vi "Read PID Kp.vi"(8 "error in (no error)":errorcluster, 10 "node":u8, 11 "ProPar in":refnum<class "PL Bronkhorst ProPar.lvclass">) -> (0 "error out":errorcluster, 2 "PID Kp":sgl, 3 "ProPar out":refnum<class "PL Bronkhorst ProPar.lvclass">)   [LabVIEW 2015, in "PL Bronkhorst ProPar.lvclass"]
doc: "Reads PID controller proportional term of the specified <b>node</b>."
uses:
  PL Bronkhorst ProPar.lvclass
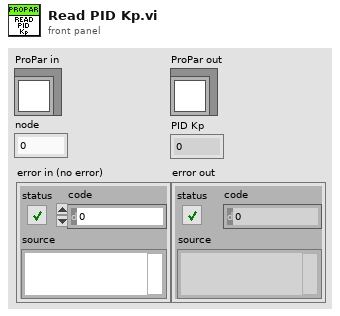
[diagram p1: front panel]
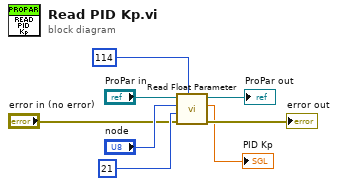
[diagram p0: block diagram]
diagram:
  n1 = call "Read Float Parameter.vi"("process number"=u8 114, "error in (no error)"="error in (no error)", "parameter number"=u8 21 ("process number"), "node"="node", "ProPar in"="ProPar in") -> ("error out"=→"error out":errorcluster, "value"=→"PID Kp":sgl, "ProPar out"=→"ProPar out":refnum<class "PL Bronkhorst ProPar.lvclass">)  [unwired: 4 in]
